vi "Cannon RPM Set.vi"(10 "Set Point RPM":dbl, 11 "EncoderDevRef":T1={"DevStatus"={"status"=FALSE, "code"=0, "source"=""}, "EncoderIndex"=enum."Invalid", "CounterIndex"=enum."Ctr 1", "DistancePerCount"=2.0, "Decoding Type"=enum."4x"}) -> (2 "READY!":bool, 3 "Vbus Out":dbl)   [LabVIEW 2012]
uses:
  <vilib>/Rock Robotics/WPI/Encoder/WPI_EncoderDevRef.ctl
  <vilib>/Rock Robotics/SystemInterfaces/Encoder/FPGA_EncoderIdx.ctl
  <vilib>/Rock Robotics/SystemInterfaces/Counter/FPGA_CounterCtrSystemIndex.ctl
  <vilib>/Rock Robotics/WPI/Encoder/WPI_EncoderType.ctl
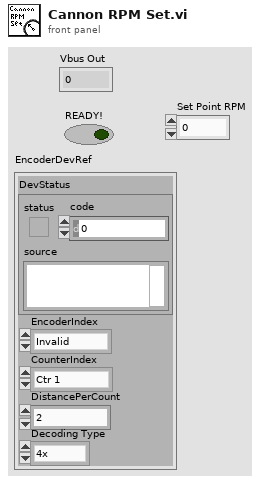
[diagram p1: front panel]
types:
  T1 = typedef "WPI_EncoderDevRef.ctl" = cluster{"DevStatus":errorcluster, "EncoderIndex":T2, "CounterIndex":T3, "DistancePerCount":dbl, "Decoding Type":T4}
  T2 = typedef "FPGA_EncoderIdx.ctl" = enum8{"Enc 0", "Enc 1", "Enc 2", "Enc 3", "Invalid"}
  T3 = typedef "FPGA_CounterCtrSystemIndex.ctl" = enum8{"Ctr 0", "Ctr 1", "Ctr 2", "Ctr 3", "Ctr 4", "Ctr 5", "Ctr 6", "Ctr 7", "Invalid"}
  T4 = typedef "WPI_EncoderType.ctl" = enum16{"1x", "2x", "4x"}
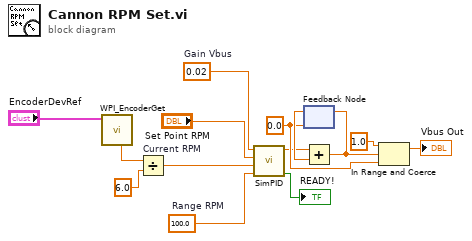
[diagram p0: block diagram]
diagram:
  w8 = 0.0
  w5 = 0.02  # Gain Vbus
  w3 = 100.0  # Range RPM
  n1 = call <vilib>:"WPI_EncoderGet.vi"("EncoderDevRef"="EncoderDevRef") -> ("Rate"=w14:dbl)  [unwired: 5 in, 5 out]
  n2 = Divide "Current RPM"(x=w14, y=6.0) -> (x/y=w12:dbl)
  n3 = call "SimPID.vi"("Range"=w3, "Position"=w12, "Set Point"="Set Point RPM", "Gain"=w5) -> ("On Target"=→"READY!":bool, "result"=w7:dbl)  [unwired: 5 in]
  n4 = feedback #1(w8) -> (w11:dbl)
  n5 = Add(x=w7, y=w11) -> (x+y=w10:dbl)
  n6 = feedback-in #1(w10) -> ()
  n7 = In Range and Coerce(upper limit=1.0, x=w10, lower limit=w8) -> (coerced(x)=→"Vbus Out":dbl)  [unwired: 1 out]
